vi "disable.vi"(8 "error in (no error)":errorcluster, 11 "Radio in":refnum<class "Radio.lvclass">) -> (0 "error out":errorcluster, 3 "Radio out":refnum<class "Radio.lvclass">)   [LabVIEW 2017, in "Radio.lvclass"]
uses:
  Radio.lvclass
  Radio.lvclass/Radio.ctl
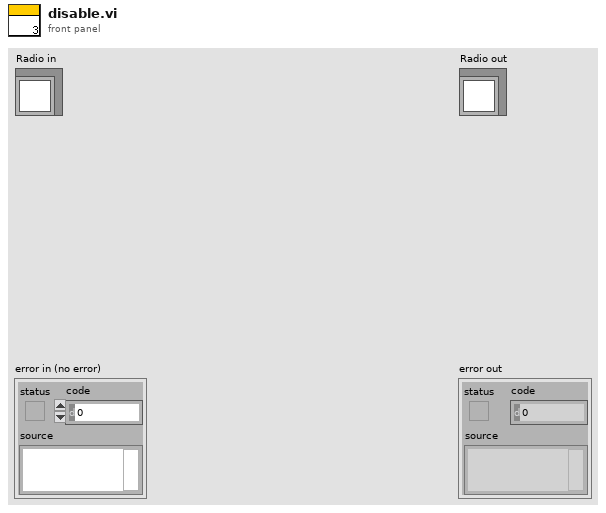
[diagram p1: front panel]
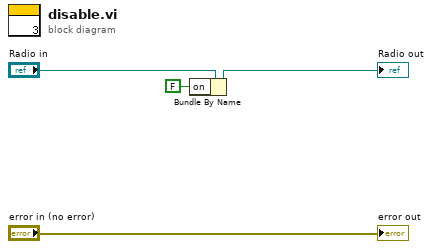
[diagram p0: block diagram]
diagram:
  n1 = Bundle By Name(cluster="Radio in", "on"=FALSE) -> (→"Radio out":refnum<class "Radio.lvclass">)
  "error out" <- "error in (no error)"
